vi "Stop Core.vi"(10 "final error code":i32, 11 "Response Matcher in":refnum<class "Response Matcher.lvclass">) -> (3 "Response Matcher out":refnum<class "Response Matcher.lvclass">)   [LabVIEW 2020, in "CANopen.lvlib" / "Response Matcher.lvlib" / "Response Matcher.lvclass"]
doc: "<p>(<strong>Filename</strong>: <span class=\"dnl\">Actor Framework.lvlib:Actor.lvclass:Stop Core.vi</span>)</p>\n<p>Defines what the actor does before it stops. Use the <strong>final error code</strong> input to determine whether the actor shut down in response to an error.</p>\n<p>By default, this method passes the Stop message along to all <a href=\"nihelplauncher://docs/csh?context=lvcore_lvcomm_af_launch_nested_actor\">auto-stop nested actors</a>. A descendant class may override this method to define additional behavior, such as shutting down any processes the actor initiated in its override of the <a href=\"nihelplauncher://docs/csh?context=lvcore_lvcomm_af_actor_core\">Actor Core</a> method.</p>"
uses:
  Response Matcher.lvclass
  Response Matcher.lvclass/Response Matcher.ctl
  <vilib>/ActorFramework/Actor/Actor.lvclass
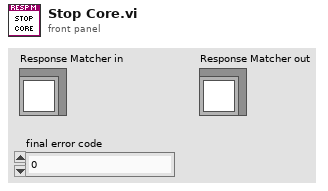
[diagram p1: front panel]
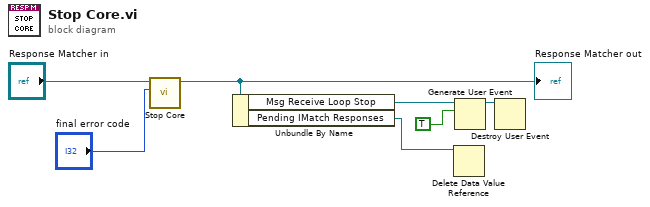
[diagram p0: block diagram]
diagram:
  n1 = call-parent "Stop Core.vi"("final error code"="final error code", "Actor in"="Response Matcher in") -> ("Actor out"=w5:refnum<class "Response Matcher.lvclass">)  [unwired: 9 in]
  "Response Matcher out" <- w5
  n2 = Unbundle By Name(w5) -> ("Msg Receive Loop Stop"=w4:refnum<user-event>, "Pending IMatch Responses"=w1:refnum<data-value>)
  n3 = Delete Data Value Reference(data value reference=w1) -> ()  [unwired: 1 in, 2 out]
  n4 = Generate User Event(user event=w4, event data cluster=TRUE ("event data")) -> (user event out=w3:refnum<user-event>)  [unwired: 2 in, 1 out]
  n5 = Destroy User Event(user event=w3) -> ()  [unwired: 1 in, 1 out]
